vi "Periodic trigger.vi"(3 "Period (s)":dbl) -> (1 "Trigger":bool)   [LabVIEW 2021]
doc: "Real-time periodic trigger."
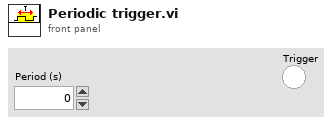
[diagram p1: front panel]
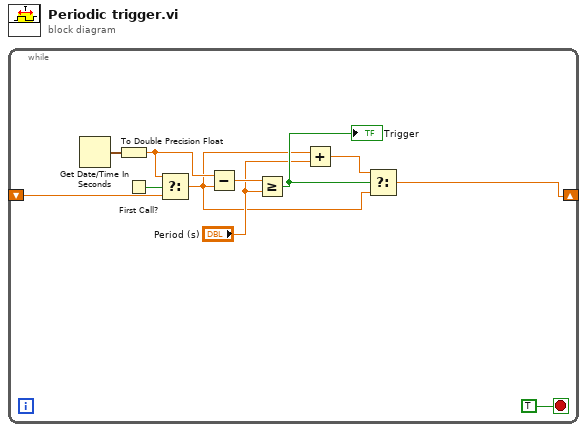
[diagram p0: block diagram]
diagram:
  n1 = while {
    shift-right: [w8] -> _
    shift-left: _ -> [w10]
    stop <- TRUE stop-if-true
    n2 = Get Date/Time In Seconds() -> (seconds since 1Jan1904=w11:timestamp)
    n3 = To Double Precision Float(number=w11) -> (double precision float=w9:dbl)
    n4 = First Call?() -> (First Call?: T/F=w5:bool)
    n5 = Select(t=w9, s=w5, f=w10) -> (s? t:f=w2:dbl)
    n6 = Subtract(x=w9, y=w2) -> (x-y=w6:dbl)
    n7 = Greater Or Equal?(x=w6, y="Period (s)") -> (x >= y?=w4:bool)
    "Trigger" <- w4
    n8 = Add(x=w2, y="Period (s)") -> (x+y=w1:dbl)
    n9 = Select(t=w1, s=w4, f=w2) -> (s? t:f=w8:dbl)
  }
